vi "Dual_Joy_Comb.vi"(7 "Rotation":bool, 10 "Joy2":dbl, 11 "Joy1":dbl) -> (3 "Output":dbl)   [LabVIEW 2017]
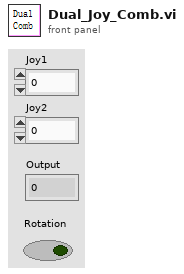
[diagram p1: front panel]
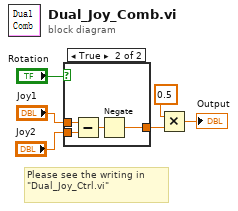
[diagram p0: block diagram]
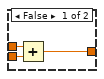
[diagram p2: hidden frame]
diagram:
  # "Please see the writing in\n\"Dual_Joy_Ctrl.vi\""
  n1 = case shown="True" "Rotation" {
    tunnel: "Joy1" -> [w8 w13]
    tunnel: "Joy2" -> [w9 w12]
    tunnel: [w7 w10] -> w2
    frame False {
      n2 = Add(x=w8, y=w9) -> (x+y=w7:dbl)
    }
    frame True {
      n3 = Subtract(x=w13, y=w12) -> (x-y=w11:dbl)
      n4 = Negate(x=w11) -> (-x=w10:dbl)
    }
  }
  n5 = Multiply(x=0.5, y=w2) -> (x*y=→"Output":dbl)
